vi "Thingworx_Example1.vi"() -> ()   [LabVIEW 2016]
panel:
  in  "stop":bool
  in  "PWM":dbl(slide) scale=0.0..255.0
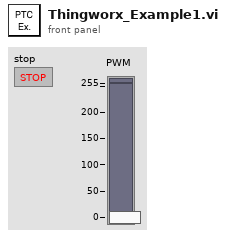
[diagram p1: front panel]
types:
  T1 = cluster{"Thing":string, "property":string, "type":string, string}
  T2 = typedef "Device.ctl" = cluster{"Name":string, "BaseURL":string, "AppKey":string, "Headers":string[], "Timeout":i32, "Identifier":string, "Password":string, "Comments":string, "Handle":u32, "# Handles":i32}
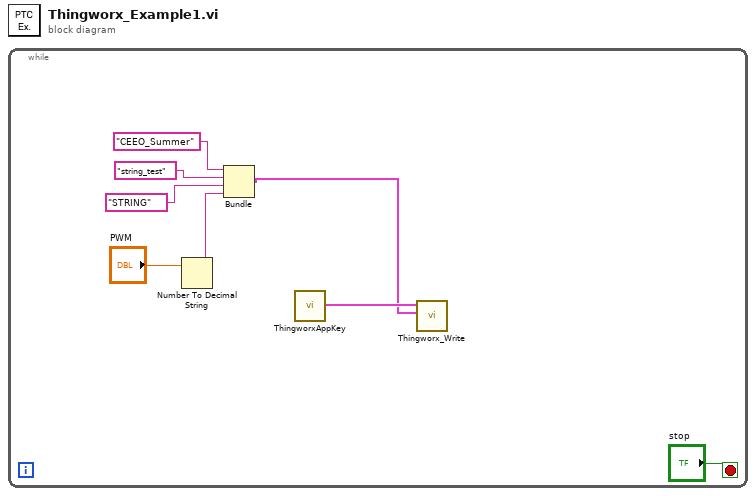
[diagram p0: block diagram]
diagram:
  n1 = while {
    stop <- "stop" stop-if-true
    n2 = Number To Decimal String(number="PWM") -> (decimal integer string=w3:string)  [unwired: 1 in]
    n3 = Bundle("Thing"="CEEO_Summer", "property"="string_test", "type"="STRING", w3) -> (w4:T1)  [unwired: 1 in]
    n4 = call "ThingworxAppKey.vi"() -> ("Device Out"=w8:T2)  [unwired: 11 in]
    n5 = call "Thingworx_Write.vi"("Property In"=w4, "Device in"=w8) -> ()  [unwired: 7 in, 3 out]
  }
